vi "struct_ads_vol_dw_dT_pTpsatRho.vi"(0 "Reference working pair (Input)":i64, 1 "Saturation pressure in Pa (Input)":dbl, 2 "Temperature in K (Input)":dbl, 3 "Pressure Pa (Input)":dbl, 5 "Der. of saturation pressure wrt. temperature in Pa/K (Input)":dbl, 7 "Density of adsorpt in kg/m3 (Input)":dbl, 9 "Der. of density of adsorpt wrt. temperature in kg/m3/K (Input)":dbl, 11 "Error (Input)":errorcluster) -> (4 "Der. of loading wrt. temperature in kg/kg/K (Output)":dbl, 15 "Error (Output)":errorcluster caption="Error(Output)")   [LabVIEW 2017]
doc: "ads_vol_dw_dT_pTpsatRho:\n * ------------------------\n *\n * Calculates derivative of equilibrium loading dw_dp with respect to\n * temperature in kg/kg/K depending on equilibrium pressure p in Pa, equilibrium\n * temperature T in K, saturation pressure p_Sat in Pa, density of adsorpt\n * rho in kg/m³, derivative of saturation pressure with respect to temperature\n * dp_sat_dT in Pa/K and derivative of density of adsorpt with respect to\n * temperature drho_dT in kg/m³/K.\n *\n * Parameters:\n * -----------\n * double p_Pa:\n * Equilibrium pressure in Pa.\n * double T_K:\n * Equilibrium temperature in K.\n * double p_sat_Pa:\n * Saturation pressure in Pa.\n * double rho_kgm3:\n * Density of adsorpt in kg/m³.\n * double dp_sat_dT_PaK:\n * Derivative of saturation pressure wrt. temperature in Pa/K.\n * double drho_dT_kgm3K:\n * Derivative of density of adsorpt wrt. temperature in kg/m³/K.\n * struct *WorkingPair:\n * Pointer of WorkingPair-struct.\n *\n * Returns:\n * --------\n * double:\n * Derivative of equilibrium loading wrt. temperature in kg/kg/K.\n *\n * Remarks:\n * --------\n * This function is only valid for isotherm models based on the volumetric\n * approach.\n *\n * History:\n * --------\n * 07/07/2021, by Jannik Driesel (supervised by Mirko Engelpracht):\n * First implementation."
uses:
  data/win32bit/libsorpPropLib.dll
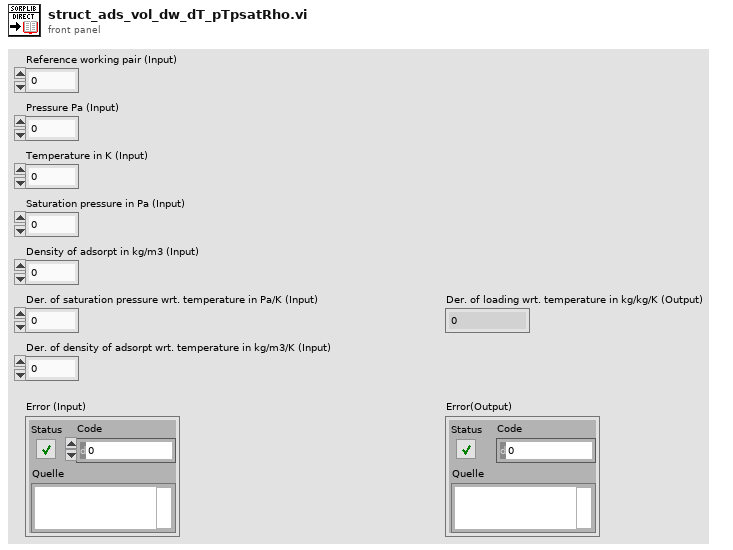
[diagram p1: front panel]
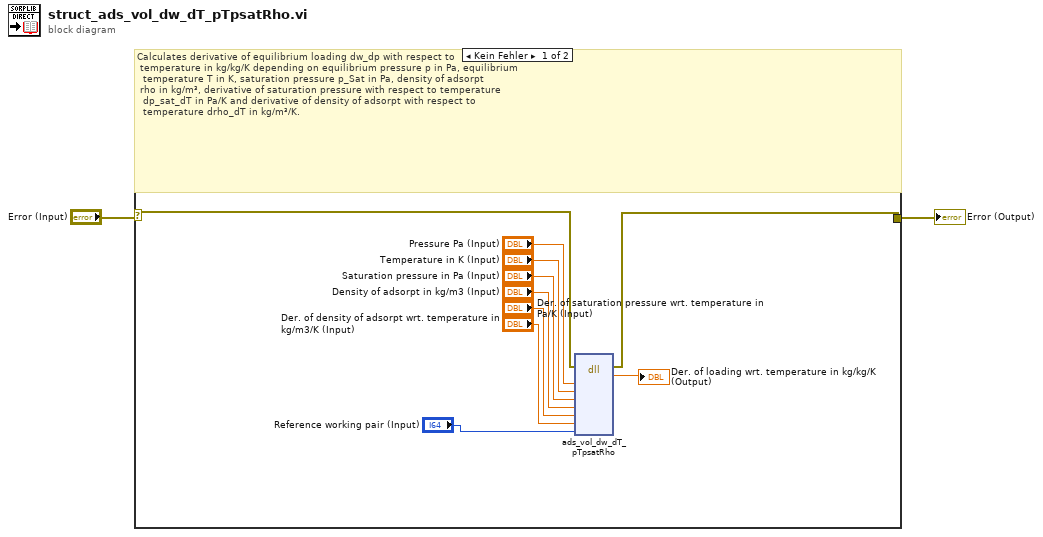
[diagram p0: block diagram]
diagram:
  n1 = case shown="Kein Fehler" "Error (Input)" {
    selector: "Error (Input)" -> [w11 w13]
    tunnel: [w10 w13] -> w1
    frame No Error {
      # "Calculates derivative of equilibrium loading dw_dp with respect to\n temperature in kg/kg/K depending on equilibrium pressure p in Pa, equilibrium\n  temperature T in K, saturation pressure p_Sat in Pa, density of adsorpt\n rho in kg/m³, derivative of saturation pressure with respect to temperature\n  dp_sat_dT in Pa/K and derivative of density of adsorpt with respect to\n  temperature drho_dT in kg/m³/K."
      n2 = dll-call lib="D:/Driesel/SorpLibLocal/LabVIEW_wrapper/data/win32bit/libsorpPropLib.dll" fn="ads_vol_dw_dT_pTpsatRho"(error in=w11, "p_Pa"="Pressure Pa (Input)", "T_K"="Temperature in K (Input)", "p_sat_Pa"="Saturation pressure in Pa (Input)", "rho_kgm3"="Density of adsorpt in kg/m3 (Input)", "dp_sat_dT_PaK"="Der. of saturation pressure wrt. temperature in Pa/K (Input)", "drho_dT_kgm3K"="Der. of density of adsorpt wrt. temperature in kg/m3/K (Input)", "workingPair"="Reference working pair (Input)") -> (error out=w10:errorcluster, "dw_dT_kgkgK"=→"Der. of loading wrt. temperature in kg/kg/K (Output)":dbl)  [unwired: 9 in, 1 out]
    }
    frame Error {
      # "Error - No calculations"
    }
  }
  "Error (Output)" <- w1
